vi "Initialize.vi"(8 "error in (no error)":errorcluster, 9 "My Helper in":refnum<class "Panel Helper.lvclass">, 10 "VI Refnum":refnum<vi>, 11 "Panel In":refnum<class "Panel.lvclass">) -> (0 "error out":errorcluster, 1 "My Helper out":refnum<class "Panel Helper.lvclass">, 3 "Panel Out":refnum<class "Panel.lvclass">)   [LabVIEW 2023, in "Panel Actor.lvlib" / "Panel.lvlib" / "Panel.lvclass"]
doc: "Inititalizes the Panel.\n\nNote: Initialization only shows the panel if the \"Auto-show\" parameter is TRUE.\n\n<B>Panel In:</B> Panel object to initialize\n<B>VI Refnum:</B> VI reference to use for initializing the Panel. Default is caller.\n<B>My Helper In:</B> Uses an existing Panel Helper object.\n<B>Error In:</B> Describes error conditions that occur before this node runs.\n\n<B>Panel Out:</B> Panel object out\n<B>My Helper Out:</B> Returns the Panel Helper object that was actually used\n<B>Error Out:</B> Contains error information.\n\n----\nPlease see the following web address for additional documentation and tutorial information:\nhttp://www.mooregoodideas.com/mgi-panel-manager/\n\nAuthor: Derek Trepanier\n\nCopyright (c) 2018, Moore Good Ideas, Inc.\n\nAll rights reserved.\n\nRedistribution and use in source and binary forms, with or without modification, are permitted provided that the following conditions are met:\n\n * Redistributions of source code must retain the above copyright notice, this list of conditions and the following disclaimer.\n * Redistributions in binary form must reproduce the above copyright notice, this list of conditions and the following disclaimer in the documentation and/or other materials provided with the distribution.\n * Neither the name of Moore Good Ideas, Inc. nor the names of its contributors may be used to endorse or promote products derived from this software without specific prior written permission.\n\nTHIS SOFTWARE IS PROVIDED BY THE COPYRIGHT HOLDERS AND CONTRIBUTORS \"AS IS\" AND ANY EXPRESS OR IMPLIED WARRANTIES, INCLUDING, BUT NOT LIMITED TO, THE IMPLIED WARRANTIES OF MERCHANTABILITY AND FITNESS FOR A PARTICULAR PURPOSE ARE DISCLAIMED. IN NO EVENT SHALL THE COPYRIGHT OWNER OR CONTRIBUTORS BE LIABLE FOR ANY DIRECT, INDIRECT, INCIDENTAL, SPECIAL, EXEMPLARY, OR CONSEQUENTIAL DAMAGES (INCLUDING, BUT NOT LIMITED TO, PROCUREMENT OF SUBSTITUTE GOODS OR SERVICES; LOSS OF USE, DATA, OR PROFITS; OR BUSINESS INTERRUPTION) HOWEVER CAUSED AND ON ANY THEORY OF LIABILITY, WHETHER IN CONTRACT, STRICT LIABILITY, OR TORT (INCLUDING NEGLIGENCE OR OTHERWISE) ARISING IN ANY WAY OUT OF THE USE OF THIS SOFTWARE, EVEN IF ADVISED OF THE POSSIBILITY OF SUCH DAMAGE."
uses:
  Panel.lvclass
  Panel Helper/Panel Helper.lvclass
  Panel.lvclass/Panel.ctl
  <vilib>/Utility/error.llb/Error Cluster From Error Code.vi
  <vilib>/ErrorRing/Error Ring.xnode
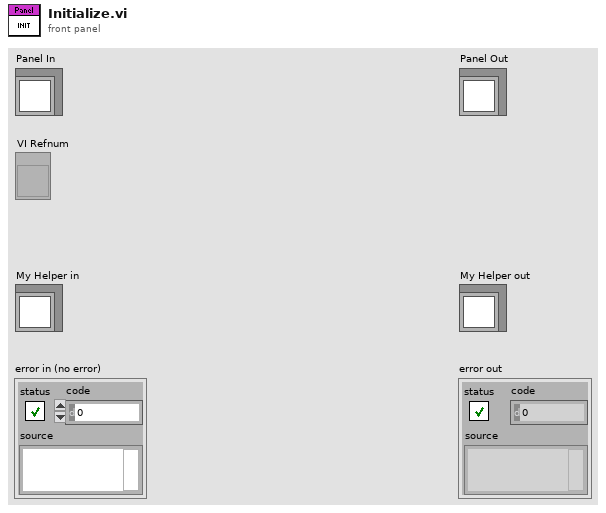
[diagram p1: front panel]
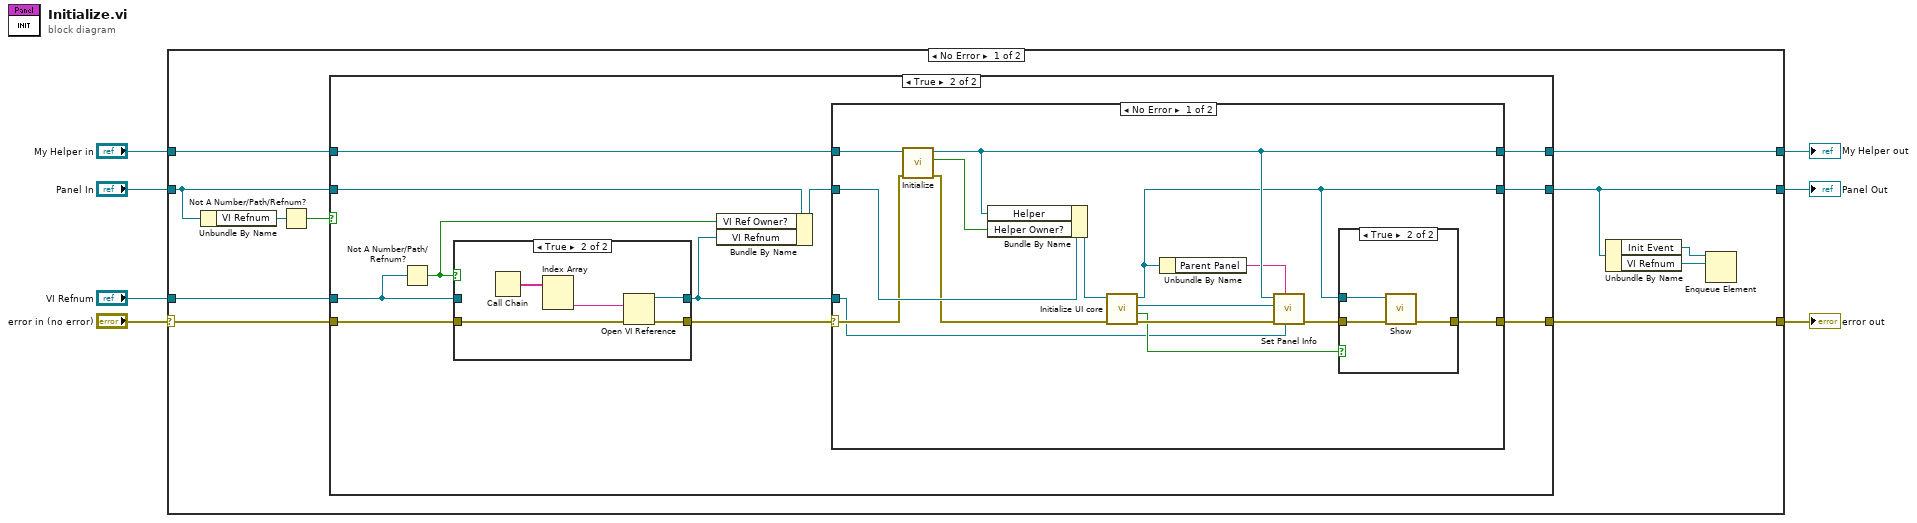
[diagram p0: block diagram]
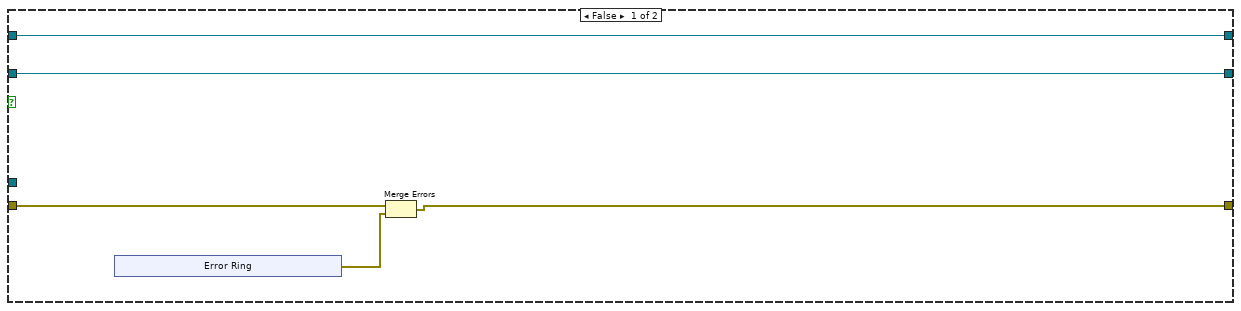
[diagram p2: hidden frame]
diagram:
  n1 = case shown="No Error" "error in (no error)" {
    selector: "error in (no error)" -> [w17 w71]
    tunnel: [w18 w71] -> w6
    tunnel: [w10 w70] -> w1
    tunnel: "Panel In" -> [w13 w70]
    tunnel: "VI Refnum" -> [w16 _]
    tunnel: "My Helper in" -> [w15 w69]
    tunnel: [w14 w69] -> w2
    frame No Error {
      n2 = Unbundle By Name(w13) -> ("VI Refnum"=w12:refnum<vi>)
      n3 = Not A Number/Path/Refnum?(number/path/refnum=w12) -> (NaN/Path/Refnum?=w11:bool)
      n4 = case shown="True" w11 {
        tunnel: [w20 w39] -> w18
        tunnel: w17 -> [w21 w38]
        tunnel: w16 -> [_ w37]
        tunnel: [w22 w36] -> w10
        tunnel: w13 -> [w22 w35]
        tunnel: w15 -> [w23 w33]
        tunnel: [w23 w32] -> w14
        frame False {
          n5 = xnode "Error Ring"() -> ("error out"=w19:errorcluster)
          n6 = Merge Errors(w21, w19) -> (w20:errorcluster)
        }
        frame True {
          n7 = Not A Number/Path/Refnum?(number/path/refnum=w37) -> (NaN/Path/Refnum?=w29:bool)
          n8 = case shown="True" w29 {
            tunnel: w38 -> [w62 w66]
            tunnel: [w62 w65] -> w34
            tunnel: [w63 w64] -> w30
            tunnel: w37 -> [w63 _]
            frame False {
            }
            frame True {
              n9 = Call Chain() -> (call chain=w68:string[])
              n10 = Index Array(array=w68) -> (element #2=w67:string)  [unwired: 2 in, 1 out]
              n11 = Open VI Reference(vi path=w67, error in (no error)=w66) -> (vi reference=w64:refnum<vi>, error out=w65:errorcluster)  [unwired: 4 in]
            }
          }
          n12 = Bundle By Name(cluster=w35, "VI Ref Owner?"=w29, "VI Refnum"=w30) -> (w31:refnum<class "Panel.lvclass">)
          n13 = case shown="No Error" w34 {
            selector: w34 -> [w49 w61]
            tunnel: [w53 w61] -> w39
            tunnel: [w41 w60] -> w36
            tunnel: w30 -> [w42 _]
            tunnel: w31 -> [w54 w60]
            tunnel: w33 -> [w51 w59]
            tunnel: [w43 w59] -> w32
            frame No Error {
              n14 = call "Initialize.vi"("error in (no error)"=w49, "Panel Helper in"=w51) -> ("error out"=w48:errorcluster, "Created New?"=w46:bool, "Panel Helper out"=w43:refnum<class "Panel Helper.lvclass">)  [unwired: 7 in]
              n15 = Bundle By Name(cluster=w54, "Helper"=w43, "Helper Owner?"=w46) -> (w47:refnum<class "Panel.lvclass">)
              n16 = call-dynamic "Initialize UI core.vi"("error in (no error)"=w48, "Panel in"=w47) -> ("error out"=w50:errorcluster, "Autoshow?"=w44:bool, "Panel Updater"=w45:refnum<class "Panel Updater.lvclass">, "Panel out"=w41:refnum<class "Panel.lvclass">)  [unwired: 6 in]
              n17 = Unbundle By Name(w41) -> ("Parent Panel"=w40:string)
              n18 = call "Set Panel Info.vi"("VI Refnum"=w42, "Parent Panel"=w40, "error in (no error)"=w50, "Panel Updater"=w45, "Panel Helper in"=w43) -> ("error out"=w52:errorcluster)  [unwired: 6 in]
              n19 = case shown="True" w44 {
                tunnel: w41 -> [_ w56]
                tunnel: w52 -> [w55 w58]
                tunnel: [w55 w57] -> w53
                frame False {
                }
                frame True {
                  n20 = call "Show.vi"("Error In"=w58, "Panel in"=w56) -> ("Error Out"=w57:errorcluster)  [unwired: 9 in]
                }
              }
            }
            frame Error {
            }
          }
        }
      }
      n21 = Unbundle By Name(w10) -> ("Init Event"=w9:refnum<queue>, "VI Refnum"=w8:refnum<vi>)
      n22 = Enqueue Element(queue=w9, element=w8) -> ()  [unwired: 2 in, 3 out]
    }
    frame Error {
    }
  }
  "error out" <- w6
  "Panel Out" <- w1
  "My Helper out" <- w2
